vi "Quit.vi"(0 "Notifier Name":string, 11 "Error In":errorcluster) -> (4 "Notifier Name Dup":string, 15 "Error Out":errorcluster)   [LabVIEW 2020]
uses:
  Spinning Disk Type Defs/SD Notifer Data.ctl
  Spinning Disk Type Defs/SD Actions.ctl
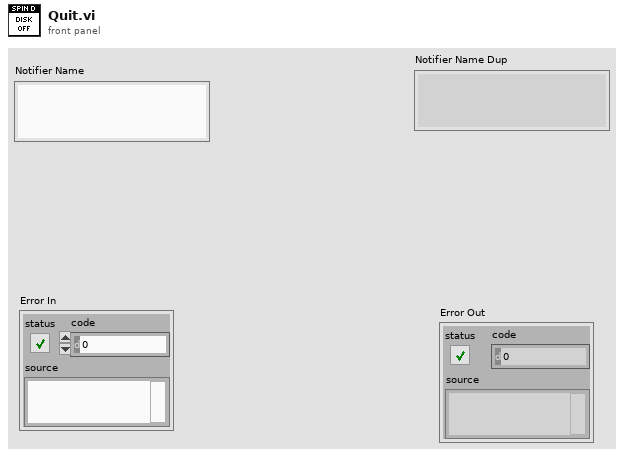
[diagram p1: front panel]
types:
  T1 = typedef "SD Notifer Data.ctl" = cluster{"Actions":T2, "Disk On?":bool, "Dichroic Pos.":i32, "Filter Wheel Pos.":i32, "Disk Pos.":i32, "Recived":bool}
  T2 = typedef "SD Actions.ctl" = enum16{"Status", "Get All Pos.", "Home All", "Set Filter Wheel Pos.", "Set Disk Pos.", "Set Dichroic Pos.", "Disk On", "Disk Off", "Quit"}
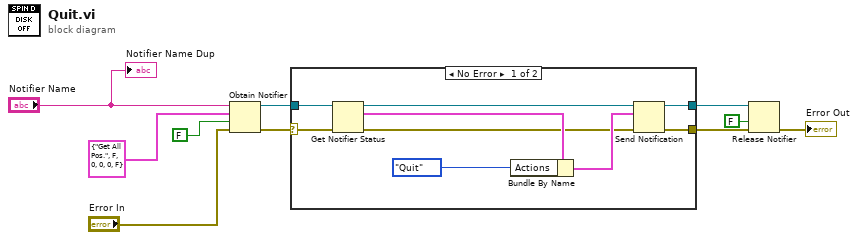
[diagram p0: block diagram]
diagram:
  n1 = Obtain Notifier(name (unnamed)="Notifier Name", notification data type=T1 {"Actions"=enum."Get All Pos.", "Disk On?"=FALSE, "Dichroic Pos."=0, "Filter Wheel Pos."=0, "Disk Pos."=0, "Recived"=FALSE} ("XLight Notifier Data"), create if not found? (T)=FALSE, error in (no error)="Error In") -> (notifier out=w6:refnum<notifier>, error out=w3:errorcluster)  [unwired: 1 out]
  n2 = case shown="No Error" w3 {
    selector: w3 -> [w18 w20]
    tunnel: w6 -> [w19 w21]
    tunnel: [w12 w21] -> w5
    tunnel: [w11 w20] -> w2
    frame No Error {
      n3 = Get Notifier Status(notifier=w19, error in (no error)=w18) -> (notifier out=w15:refnum<notifier>, current notification=w17:T1, error out=w13:errorcluster)  [unwired: 2 out]
      n4 = Bundle By Name(cluster=w17, "Actions"=SD_Actions."Quit") -> (w14:T1)
      n5 = Send Notification(notification=w14, notifier=w15, error in (no error)=w13) -> (notifier out=w12:refnum<notifier>, error out=w11:errorcluster)
    }
    frame Error {
    }
  }
  n6 = Release Notifier(notifier=w5, force destroy? (F)=FALSE, error in (no error)=w2) -> (error out=→"Error Out":errorcluster)  [unwired: 2 out]
  "Notifier Name Dup" <- "Notifier Name"
